vi "LockinDAQ.Simulate Waveguide.vi"(8 "error in (no error)":errorcluster, 9 "AO (Vsg)":waveform(dbl), 10 "AO (Vsource)":waveform(dbl), 11 "LockinDAQ":refnum<class "LockinDAQ.lvclass">) -> (0 "error out":errorcluster, 2 "AI (V)":waveform(dbl), 3 "LockinDAQ out":refnum<class "LockinDAQ.lvclass">)   [LabVIEW 2016, in "LockinDAQ.lvclass"]
uses:
  LockinDAQ.lvclass
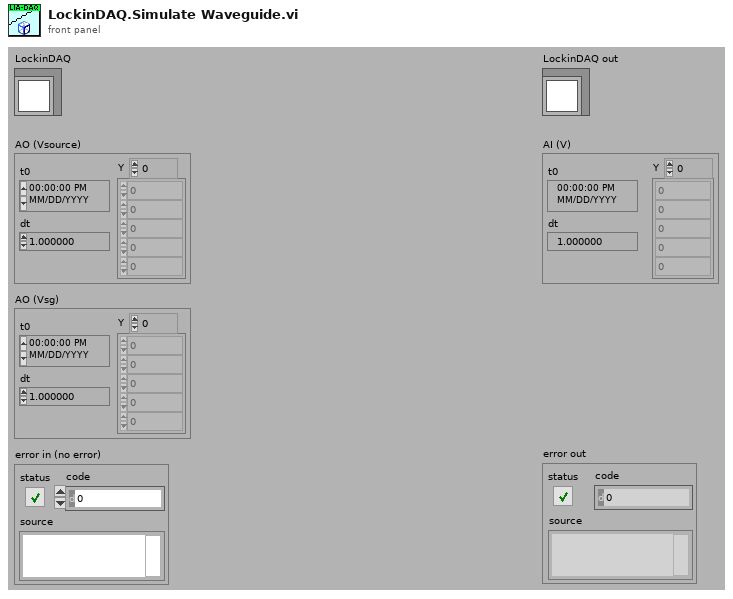
[diagram p1: front panel]
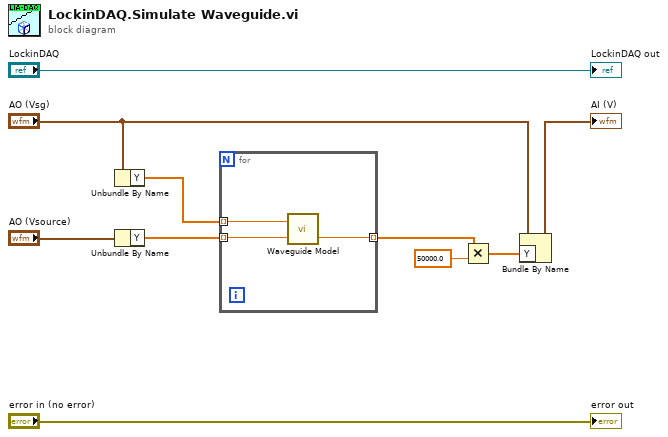
[diagram p0: block diagram]
diagram:
  n1 = Unbundle By Name("AO (Vsg)") -> ("Y"=w7:dbl[])
  n2 = Unbundle By Name("AO (Vsource)") -> ("Y"=w8:dbl[])
  n3 = for {
    tunnel: w8 -> [w13] mode=indexing
    tunnel: w7 -> [w12] mode=indexing
    tunnel: [w11] -> w4 mode=indexing
    n4 = call "Waveguide Model.vi"("Vs (V)"=w13, "Vsg (V)"=w12) -> ("I[Vsg] (A)"=w11:dbl)  [unwired: 1 out]
  }
  n5 = Multiply(x=w4, y=50000.0) -> (x*y=w3:dbl[])
  n6 = Bundle By Name(cluster="AO (Vsg)", "Y"=w3) -> (→"AI (V)":waveform(dbl))
  "error out" <- "error in (no error)"
  "LockinDAQ out" <- "LockinDAQ"
